vi "compare test.vi"() -> ()   [LabVIEW 2009]
panel:
  out "appended array":bool[](array[boolean])
  in  "Array 2":bool[](array[boolean])
  in  "Array":string[][][](array[string])
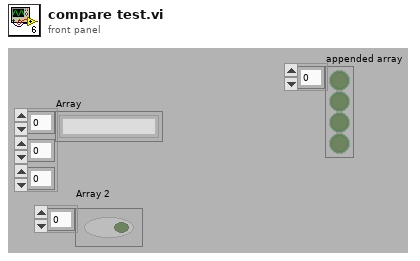
[diagram p1: front panel]
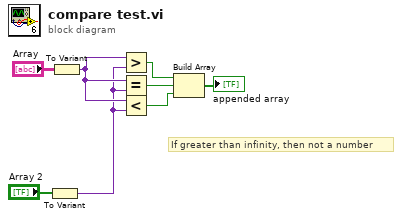
[diagram p0: block diagram]
diagram:
  # "If greater than infinity, then not a number"
  n1 = To Variant(anything="Array 2") -> (Variant=w5:variant)
  n2 = To Variant(anything="Array") -> (Variant=w6:variant)
  n3 = Greater?(x=w6, y=w5) -> (0:w4:bool)
  n4 = Equal?(x=w6, y=w5) -> (x = y?=w2:bool)
  n5 = Less?(x=w6, y=w5) -> (x < y?=w1:bool)
  n6 = Build Array(w4, w2, w1) -> (→"appended array":bool[])
